vi "Check Apps.vi"(11 "App Watcher in":refnum<class "App Watcher.lvclass">) -> ()   [LabVIEW 2020, in "PicoG-App.lvlib" / "App Watcher.lvclass"]
uses:
  App Watcher.lvclass
  App Watcher.lvclass/App Watcher.ctl
  App Update Data.ctl
  ViaApp/ViaApp.lvclass
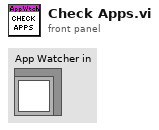
[diagram p1: front panel]
types:
  T1 = typedef "PicoG-App.lvlib/App Watcher.lvclass/Ref Data.ctl" = cluster{"App Map":map{path, refnum<class "ViaApp.lvclass">}, "App Update Event":refnum<user-event>}
  T2 = typedef "PicoG-App.lvlib/App Watcher.lvclass/App Update Data.ctl" = cluster{"App":refnum<class "ViaApp.lvclass">}
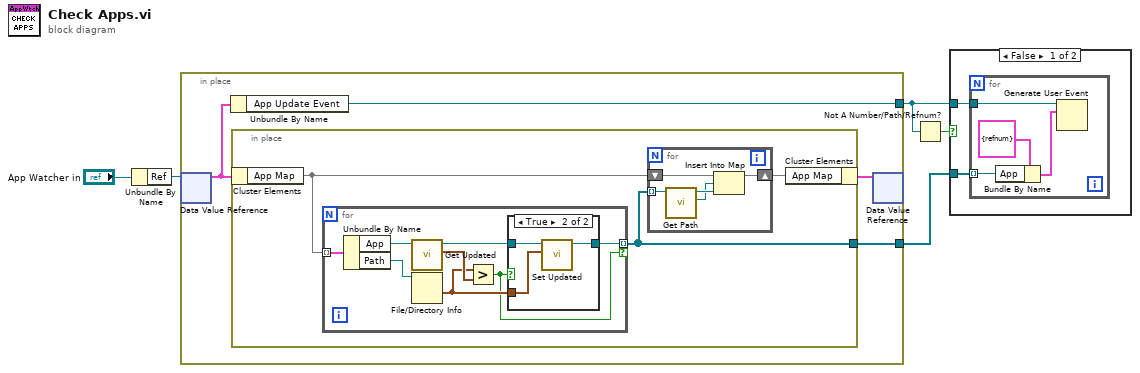
[diagram p0: block diagram]
diagram:
  n1 = Unbundle By Name("App Watcher in") -> ("Ref"=w5:refnum<data-value>)
  n2 = in-place {
    in-place-border: [w8] -> w3
    in-place-border: [w6] -> w2
    n3 = in-place-dvr #1(w5) -> (w7:T1)  [unwired: 1 out]
    n4 = Unbundle By Name(w7) -> ("App Update Event"=w6:refnum<user-event>)
    n5 = in-place {
      in-place-border: [w10] -> w8
      n6 = in-place-cluster #2(w7) -> ("App Map"=w12:map{path, refnum<class "ViaApp.lvclass">})
      n7 = for {
        tunnel: w12 -> [w25] mode=indexing
        tunnel: [w19] -> w10 mode=indexing if=w18
        n8 = Unbundle By Name(w25) -> ("App"=w23:refnum<class "ViaApp.lvclass">, "Path"=w24:path)
        n9 = call "Get Updated.vi"("ViaApp in"=w23) -> ("Last Update"=w22:timestamp, "ViaApp out"=w21:refnum<class "ViaApp.lvclass">)  [unwired: 8 in, 1 out]
        n10 = File/Directory Info(path=w24) -> (last mod=w20:timestamp)  [unwired: 1 in, 6 out]
        n11 = Greater?(x=w20, y=w22) -> (0:w18:bool)
        n12 = case shown="True" w18 {
          tunnel: w21 -> [w26 w29]
          tunnel: w20 -> [_ w28]
          tunnel: [w26 w27] -> w19
          frame False {
          }
          frame True {
            n13 = call "Set Updated.vi"("Updated"=w28, "ViaApp in"=w29) -> ("ViaApp out"=w27:refnum<class "ViaApp.lvclass">)  [unwired: 8 in, 1 out]
          }
        }
      }
      n14 = for {
        shift-right: [w16] -> w11
        shift-left: w12 -> [w17]
        tunnel: w10 -> [w13] mode=indexing
        n15 = call "Get Path.vi"("ViaApp in"=w13) -> ("Path"=w14:path, "ViaApp out"=w15:refnum<class "ViaApp.lvclass">)  [unwired: 8 in, 1 out]
        n16 = Insert Into Map(map in=w17, key=w14, value=w15) -> (map out=w16:map{path, refnum<class "ViaApp.lvclass">})  [unwired: 2 out]
      }
      n17 = in-place-cluster #2("App Map"=w11) -> (w9:T1)
    }
    n18 = in-place-dvr #1(w9) -> ()  [unwired: 2 out]
  }
  n19 = Not A Number/Path/Refnum?(number/path/refnum=w2) -> (NaN/Path/Refnum?=w1:bool)
  n20 = case shown="False" w1 {
    tunnel: w3 -> [w31 _]
    tunnel: w2 -> [w30 _]
    frame False {
      n21 = for {
        tunnel: w31 -> [w33] mode=indexing
        tunnel: w30 -> [w35]
        n22 = Bundle By Name(cluster=T2 {"App"=refnum} ("App Update Data"), "App"=w33) -> (w32:T2)
        n23 = Generate User Event(user event=w35, event data cluster=w32) -> ()  [unwired: 2 in, 2 out]
      }
    }
    frame True {
    }
  }
